vi "ButtonBoxVars.vi"() -> ()   [LabVIEW 2014]
panel:
  out "ButtonBoxOutput":bool[](array[boolean])
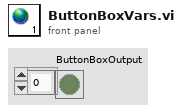
[diagram p1: front panel]
diagram:
